vi "PH_Stepmotor_BaseClass.Evt Call Axis Settings.vi"(0 "i ref in":refnum<vi>, 1 "Address":T3={"Instance"="N/A", "Motor Nr"=0}, 3 "Settings to set":T1={"Sign change"=FALSE, "Width"=0.0, "Calibration"=0.0, "Unit"="Steps", "Motor Type"=enum."Unspecific", "Unit Width"="", "Unit CF"=""} caption="Axis Settings", 5 "error in":errorcluster) -> (14 "i ref out":refnum<vi>, 19 "error out":errorcluster)   [LabVIEW 2014, in "PH_Stepmotor_BaseClass.lvlib"]
uses:
  PH_Stepmotor_BaseClass.lvlib
  PH_Stepmotor_BaseClass.Axis Address.ctl
  PH_Stepmotor_BaseClass.Axis Settings.ctl
  PH_Stepmotor_BaseClass.Motor Type.ctl
  CSCore/CSSystem/CoreLib/CoreLib.short 2 byte array.vi
  CSCore/CSSystem/CoreLib/CoreLib.string 2 byte array.vi
  CSCore/CSSystem/CoreLib/CoreLib.double 2 byte array.vi
  CSCore/CSSystem/CoreLib/CoreLib.int 2 byte array.vi
  CSCore/CSSystem/CoreLib/CoreLib.lvlib
  CSCore/BaseProcess/BaseProcess.lvlib
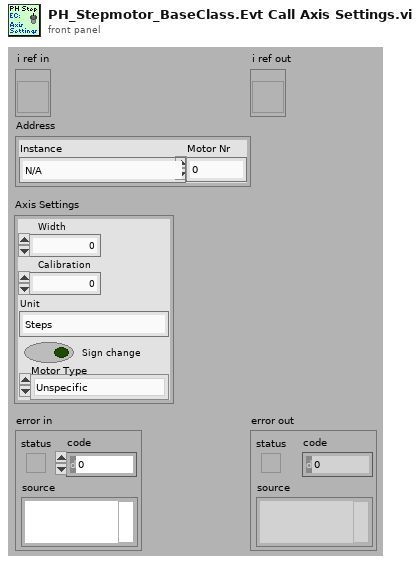
[diagram p1: front panel]
types:
  T1 = typedef "PH_Stepmotor_BaseClass.lvlib/PH_Stepmotor_BaseClass.Axis Settings.ctl" = cluster{"Sign change":bool, "Width":dbl, "Calibration":dbl, "Unit":string, "Motor Type":T2, "Unit Width":string, "Unit CF":string}
  T2 = typedef "PH_Stepmotor_BaseClass.lvlib/PH_Stepmotor_BaseClass.Motor Type.ctl" = enum16{"Unspecific", "OWIS 49.120.2633", "OWIS 49.060.1033", "OWIS 43.040.2558", "Diamond Motion 2200 series", "OWIS 49.120.266B.MV6", "Calorimeter", "Linear Stage 1", "MICOS VT-80", "MICOS VT-80 S", "Standa Rotstage nt0.95A", "PUF RA 320.200", "PUF RA 800.200", "PUF RA 800.400", "PUF RA 400.50", "1324.nn.800.50", "1324.n9c.800.50", "1324.nn.320.200", "1324.nn.400.200", "1324.nn.800.200", "1324.nn.400.50", "1324.8c9c.800.50", "1324.8c9c.400.200"}
  T3 = typedef "PH_Stepmotor_BaseClass.lvlib/PH_Stepmotor_BaseClass.Axis Address.ctl" = cluster{"Instance":string, "Motor Nr":i32}
  T4 = typedef "CoreDefs.rawDataType.ctl" = i8[]
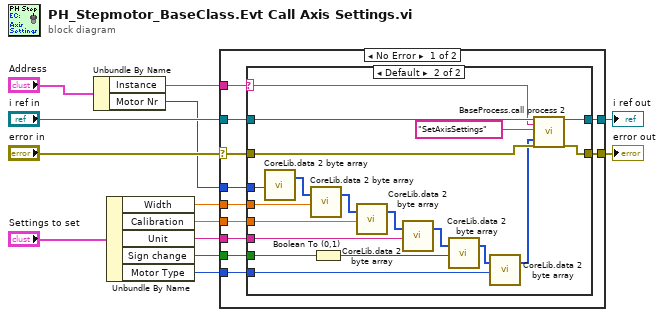
[diagram p0: block diagram]
diagram:
  n1 = Unbundle By Name("Address") -> ("Instance"=w2:string, "Motor Nr"=w1:i32)
  n2 = Unbundle By Name("Settings to set") -> ("Width"=w7:dbl, "Calibration"=w6:dbl, "Unit"=w5:string, "Sign change"=w4:bool, "Motor Type"=w3:T2)
  n3 = case shown="No Error" "error in" {
    selector: "error in" -> [w20 w46]
    tunnel: [w24 w46] -> w10
    tunnel: w2 -> [w19 _]
    tunnel: "i ref in" -> [w23 w47]
    tunnel: [w22 w47] -> w12
    tunnel: w1 -> [w21 _]
    tunnel: w5 -> [w18 _]
    tunnel: w4 -> [w17 _]
    tunnel: w6 -> [w16 _]
    tunnel: w7 -> [w15 _]
    tunnel: w3 -> [w14 _]
    frame No Error {
      n4 = case shown="Default" w19 {
        selector: w19 -> [_ w27]
        tunnel: [w26 w45] -> w24
        tunnel: w20 -> [w26 w43]
        tunnel: w23 -> [w25 w42]
        tunnel: [w25 w41] -> w22
        tunnel: w21 -> [_ w40]
        tunnel: w18 -> [_ w35]
        tunnel: w17 -> [_ w29]
        tunnel: w16 -> [_ w34]
        tunnel: w15 -> [_ w33]
        tunnel: w14 -> [_ w30]
        frame "N/A" {
        }
        frame Default {
          n5 = call-poly "CoreLib.data 2 byte array.vi"("i32"=w40) -> ("byteArray out"=w39:T4)  [unwired: 18 in]
          n6 = call-poly "CoreLib.data 2 byte array.vi"("byteArray"=w39, "f64"=w33) -> ("byteArray out"=w38:T4)  [unwired: 17 in]
          n7 = Boolean To (0,1)(Boolean=w29) -> (0, 1=w28:i16)
          n8 = call-poly "CoreLib.data 2 byte array.vi"("byteArray"=w38, "f64"=w34) -> ("byteArray out"=w37:T4)  [unwired: 17 in]
          n9 = call-poly "CoreLib.data 2 byte array.vi"("byteArray"=w37, "string"=w35) -> ("byteArray out"=w36:T4)  [unwired: 17 in]
          n10 = call-poly "CoreLib.data 2 byte array.vi"("byteArray"=w36, "i16"=w28) -> ("byteArray out"=w32:T4)  [unwired: 17 in]
          n11 = call-poly "CoreLib.data 2 byte array.vi"("byteArray"=w32, "i16"=w30) -> ("byteArray out"=w31:T4)  [unwired: 17 in]
          n12 = call "BaseProcess.call process 2.vi"("i ref in"=w42, "Object"=w27, "Selector"="SetAxisSettings", "Data"=w31, "error in (no error)"=w43) -> ("i ref out"=w41:refnum<vi>, "error out"=w45:errorcluster)  [unwired: 13 in]
        }
      }
    }
    frame Error {
    }
  }
  "i ref out" <- w12
  "error out" <- w10
